vi "Intermods.vi"() -> ()   [LabVIEW 2018]
doc: "PNA-X Example."
uses:
  Instance           1 17Saved   Intermods .vi
  PNA-X.lvlib
panel:
  out "XY Graph":cluster{"X-Axis":dbl[], "Data":dbl[]}(graph)
  out "error out":errorcluster
  in  "error in (no error)":errorcluster
  out "VISA Out":refnum<visa-resource-name>
  in  "VISA IN":refnum<visa-resource-name>
  # "1. Select Instrument Source from the \"VISA IN\" drop down.\n2. Run vi"
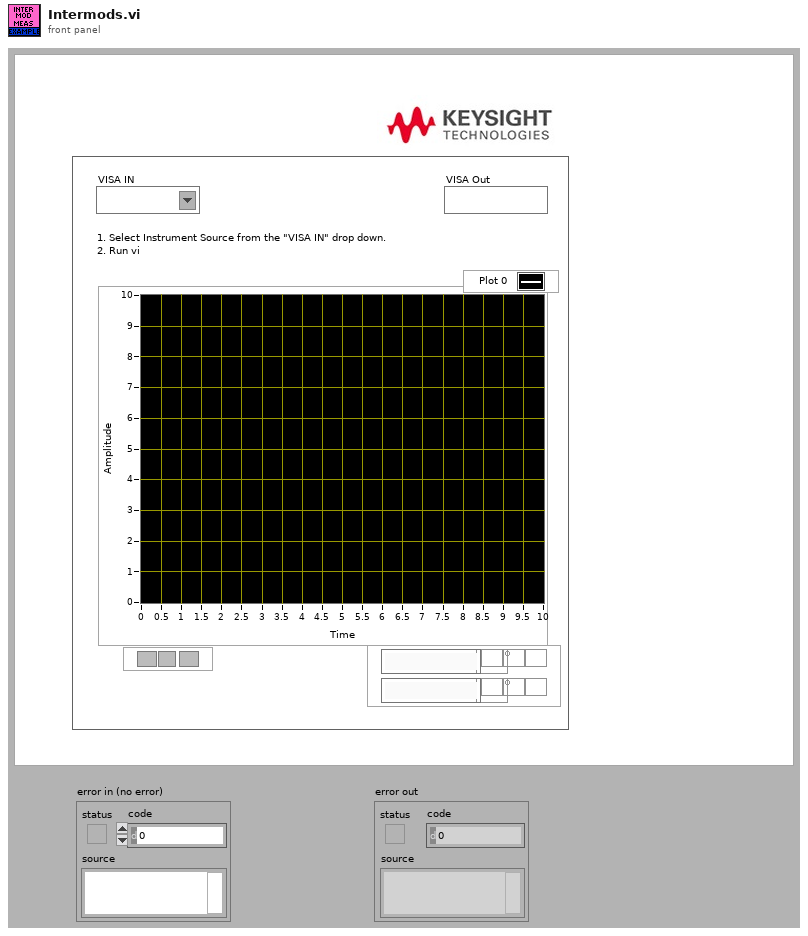
[diagram p1: front panel]
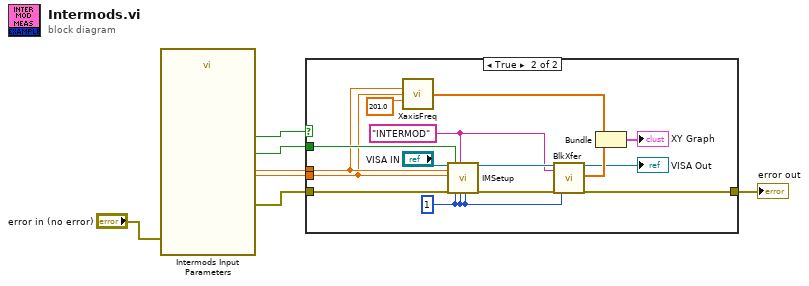
[diagram p0: block diagram]
diagram:
  n1 = call "Intermods Input Parameters"("error in (no error)"="error in (no error)") -> ("F2"=w3:dbl, "F1"=w4:dbl, "Autoscale?"=w5:bool, "Execute"=w7:bool, "error out"=w6:errorcluster)  [unwired: 14 in]
  n2 = case shown="True" w7 {
    tunnel: w6 -> [w8 w23]
    tunnel: w5 -> [_ w22]
    tunnel: w4 -> [_ w15]
    tunnel: w3 -> [_ w14]
    tunnel: [w8 w9] -> w1
    frame False {
    }
    frame True {
      w16 = "INTERMOD" ("Filename")
      w17 = 1 ("Channel")
      n3 = call "XaxisFreq.vi"("Start Frequency"=w15, "Stop Frequency"=w14, "Points"=201.0) -> ("X-Axis"=w12:dbl[])  [unwired: 12 in]
      n4 = call "IMSetup.vi"("VISA IN"="VISA IN", "F1"=w15, "F2"=w14, "error in"=w23, "Autoscale?"=w22, "Channel"=w17, "Filename"=w16, "Window"=w17, "Trace"=w17) -> ("VISA Out"=w19:refnum<visa-resource-name>, "error out"=w18:errorcluster)  [unwired: 9 in]
      n5 = call "BlkXfer.vi"("VISA IN"=w19, "FileName"=w16, "error in"=w18, "Channel"=w17) -> ("VISA Out"=→"VISA Out":refnum<visa-resource-name>, "Data"=w20:dbl[], "error out"=w9:errorcluster)  [unwired: 13 in]
      n6 = Bundle("X-Axis"=w12, "Data"=w20) -> (→"XY Graph":cluster{"X-Axis":dbl[], "Data":dbl[]})  [unwired: 1 in]
    }
  }
  "error out" <- w1
